vi "Set Config Variables.vi"(7 "LabVIEW Web Service Request":refnum<class "Web Request.lvclass">) -> ()   [LabVIEW 2015]
uses:
  <vilib>/wsapi/Web Request.lvclass
panel:
  # "Use the Web Service Request input terminal to call the VIs on the Web Services palette. Do not remove it from the connector pane unless you don't need access to the palette."
  # "Each additional control wired to the connector pane will be available as an input in the URL. To include an indicator in terminal-mode output (the default setting), it must also be wired to the connector pane."
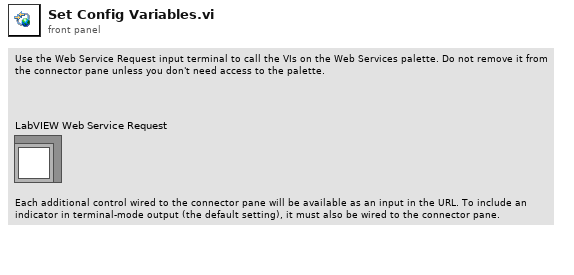
[diagram p1: front panel]
types:
  T1 = typedef "Address Book Data.lvlib/Contact.ctl" = cluster{"ID":u32, "Last Name":string, "First Name":string, "Middle Name":string, "Phone":string, "Address":T2, "Favorite?":bool}
  T2 = typedef "Address Book Data.lvlib/Address.ctl" = cluster{"Street":string, "City":string, "State":string, "Postal Code":string}
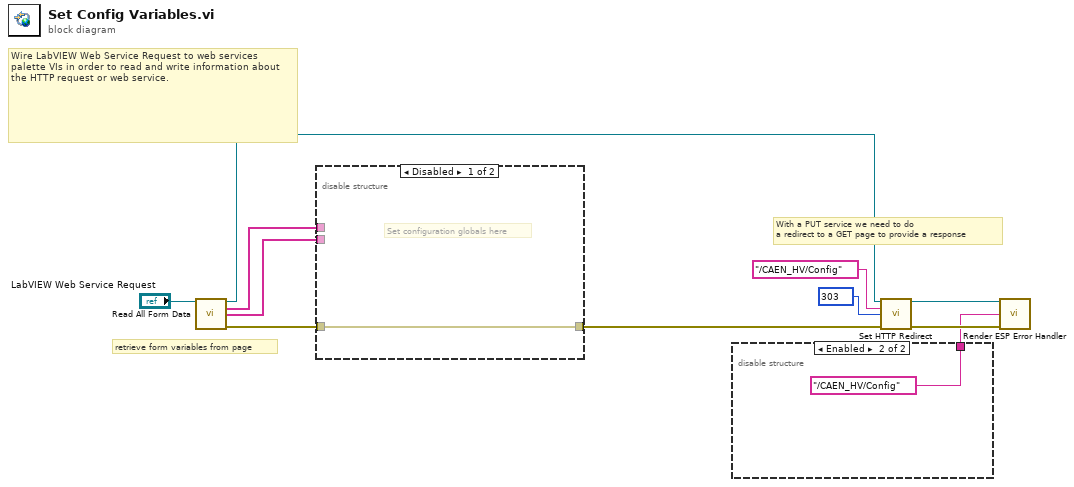
[diagram p0: block diagram]
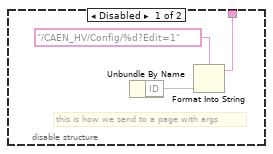
[diagram p2: hidden frame]
diagram:
  w10 = 303 items=["100"=100, "101"=101, "200"=200, "201"=201, "202"=202, "203"=203, "204"=204, "205"=205, "206"=206, "300"=300, "301"=301, "302"=302, "303"=303, "304"=304, "305"=305, "306"=306, "307"=307, "400"=400, "401"=401, "402"=402, "403"=403, "404"=404, "405"=405, "406"=406, "407"=407, "408"=408, "409"=409, "410"=410, "411"=411, "412"=412, "413"=413, "414"=414, "415"=415, "416"=416, "417"=417, "500"=500, "501"=501, "502"=502, "503"=503, "504"=504, "505"=505] ("response code (307)")
  # "retrieve form variables from page"
  # "With a PUT service we need to do\na redirect to a GET page to provide a response"
  # "Wire LabVIEW Web Service Request to web services palette VIs in order to read and write information about the HTTP request or web service."
  n1 = call <vilib>:"Read All Form Data.vi"("LabVIEW Web Service Request"="LabVIEW Web Service Request") -> ("LabVIEW Web Service Request out"=w6:refnum<class "Web Request.lvclass">, "Key"=w4:string[], "Value"=w3:string[], "error out"=w2:errorcluster)  [unwired: 10 in, 1 out]
  n2 = disable-structure shown="Disabled" {
    disable-tunnel: w4 -> [_ _]
    disable-tunnel: w3 -> [_ _]
    disable-tunnel: w2 -> [w12 _]
    disable-tunnel: [w12 _] -> w1
    frame Disabled {
      # "Set configuration globals here"
    }
    frame Enabled {
    }
  }
  n3 = disable-structure shown="Enabled" {
    disable-tunnel: [w15 "/CAEN_HV/Config" ("Link")] -> w7
    frame Disabled {
      # "this is how we send to a page with args"
      n4 = Unbundle By Name() -> (w13:T1, "ID"=w14)
      n5 = Format Into String(format string="/CAEN_HV/Config/%d?Edit=1" ("Link"), w14) -> (resulting string=w15:string)  [unwired: 2 in, 1 out]
    }
    frame Enabled {
    }
  }
  n6 = call <vilib>:"Set HTTP Redirect.vi"("LabVIEW Web Service Request"=w6, "redirect URL"="/CAEN_HV/Config", "response code (307)"=w10, "error in (no error)"=w1) -> ("LabVIEW Web Service Request out"=w8:refnum<class "Web Request.lvclass">, "error out"=w9:errorcluster)  [unwired: 10 in]
  n7 = call "Render ESP Error Handler.vi"("LabVIEW Web Service Request"=w8, "Link"=w7, "error in (no error)"=w9) -> ()  [unwired: 11 in, 2 out]
